vi "StringToBoolean.vi"(8 "error in (no error)":errorcluster, 11 "Input":string) -> (0 "error out":errorcluster, 3 "Boolean":bool)   [LabVIEW 2014]
uses:
  <vilib>/Utility/error.llb/Error Cluster From Error Code.vi
  <vilib>/ErrorRing/Error Ring.xnode
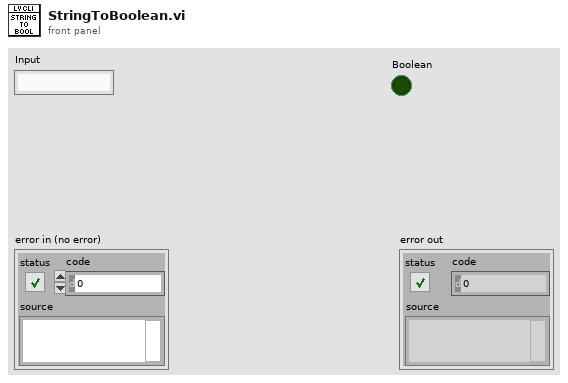
[diagram p1: front panel]
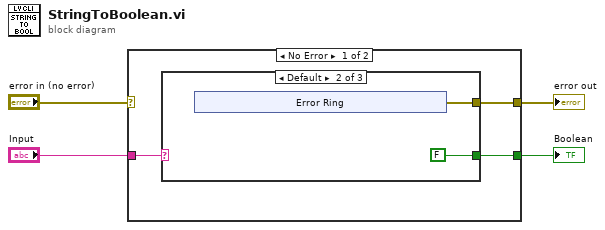
[diagram p0: block diagram]
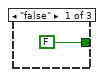
[diagram p2: hidden frame]
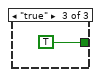
[diagram p3: hidden frame]
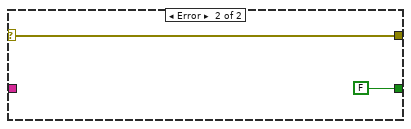
[diagram p4: hidden frame]
diagram:
  n1 = case shown="No Error" "error in (no error)" {
    selector: "error in (no error)" -> [_ w18]
    tunnel: [w7 FALSE] -> w4
    tunnel: "Input" -> [w6 _]
    tunnel: [w5 w18] -> w1
    frame No Error {
      n2 = case shown="Default" w6 {
        tunnel: [FALSE FALSE TRUE] -> w7
        tunnel: [_ w9 _] -> w5
        frame "false" {
        }
        frame Default {
          n3 = xnode "Error Ring"() -> ("error out"=w9:errorcluster)
        }
        frame "true" {
        }
      }
    }
    frame Error {
    }
  }
  "Boolean" <- w4
  "error out" <- w1
